vi "UsrProfiles-Selective save.vi"(11 "Changes array ctrl":refnum<vi>) -> (0 "error out":errorcluster)   [LabVIEW 2017]
uses:
  Typedefs/Which path.ctl
  <vilib>/Utility/config.llb/NI_LVConfig.lvlib
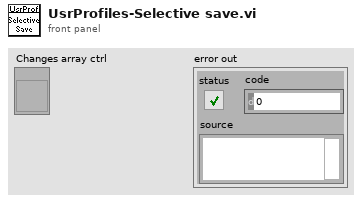
[diagram p1: front panel]
types:
  T1 = typedef "Changes info cluster-DBL.ctl" = cluster{"Section names":string[], "Keys data":T2}
  T2 = typedef "Ini file interface (DBL).ctl" = cluster{"key":string, "Save?":bool, "Default":dbl}[]
  T3 = typedef "Changes info cluster-STRING.ctl" = cluster{"Section names":string[], "Keys data":T4}
  T4 = typedef "Ini file interface (String).ctl" = cluster{"key":string, "Save?":bool, "Default":string}[]
  T5 = typedef "Changes info cluster-BOOL.ctl" = cluster{"Section names":string[], "Keys data":T6}
  T6 = typedef "Ini file interface (Boolean).ctl" = cluster{"key":string, "Save?":bool, "Default":bool}[]
  T7 = typedef "Which path.ctl" = enum16{"Configuration Files", "Calibration Files", "Images", "Setup.ini", "Loaded User profile.ini", "User's-Previous session.ini", "New user profile.ini", "Selected User profile.ini", "User profiles folder", "Power meter scaling.txt", "FOV Cal.ini"}
  T8 = typedef "NI_LVConfig.lvlib/Config Data RefNum.ctl" = refnum<k1>
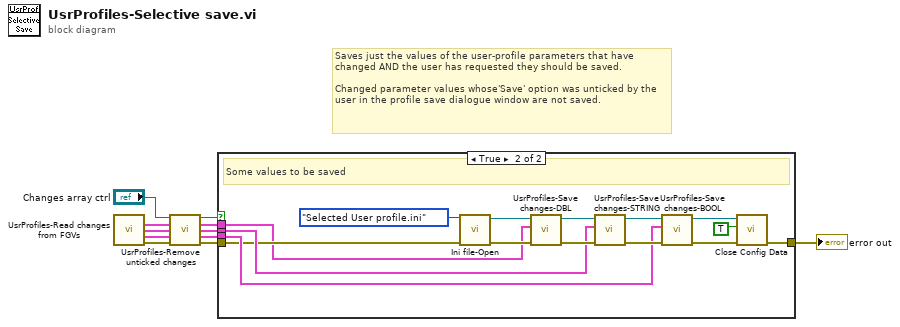
[diagram p0: block diagram]
diagram:
  # "Saves just the values of the user-profile parameters that have changed AND the user has requested they should be saved.\n\nChanged parameter values whose'Save' option was unticked by the user in the profile save dialogue window are not saved."
  n1 = call "UsrProfiles-Read changes from FGVs.vi"() -> ("Keys of changed parameters-DBL"=w9:T1, "Keys of changed parameters-STRING"=w8:T3, "Keys of changed parameters-BOOL"=w7:T5, "error out"=w11:errorcluster)  [unwired: 10 in, 2 out]
  n2 = call "UsrProfiles-Remove unticked changes.vi"("Changes array ctrl"="Changes array ctrl", "Keys of changed parameters-DBL"=w9, "Keys of changed parameters-STRING"=w8, "Keys of changed parameters-BOOL"=w7, "error in (no error)"=w11) -> ("Some values to be saved"=w2:bool, "Keys of changed parameters-DBL"=w3:T1, "Keys of changed parameters-STRING"=w6:T3, "Keys of changed parameters-BOOL"=w5:T5, "error out"=w4:errorcluster)  [unwired: 6 in]
  n3 = case shown="True" w2 {
    tunnel: w6 -> [_ w18]
    tunnel: w5 -> [_ w17]
    tunnel: [w12 w16] -> w1
    tunnel: w4 -> [w12 w14]
    tunnel: w3 -> [_ w13]
    frame False {
      # "No values to be saved"
    }
    frame True {
      # "Some values to be saved"
      n4 = call "Ini file-Open.vi"("Error In"=w14, "Which file?"=Which_path."Selected User profile.ini" ("Which file? (User profile.ini)")) -> ("error out"=w15:errorcluster, "User profile ini file ref"=w25:T8)  [unwired: 6 in, 2 out]
      n5 = call "UsrProfiles-Save changes-DBL.vi"("error in (no error)"=w15, "Keys of changed parameters-DBL"=w13, "User profile ini file ref"=w25) -> ("error out"=w21:errorcluster, "User profile ini file ref"=w24:T8)  [unwired: 7 in]
      n6 = call "UsrProfiles-Save changes-STRING.vi"("error in (no error)"=w21, "Keys of changed parameters-STRING"=w18, "User profile ini file ref"=w24) -> ("error out"=w22:errorcluster, "User profile ini file ref"=w23:T8)  [unwired: 7 in]
      n7 = call "UsrProfiles-Save changes-BOOL.vi"("error in (no error)"=w22, "Keys of changed parameters-BOOL"=w17, "User profile ini file ref"=w23) -> ("error out"=w19:errorcluster, "User profile ini file ref"=w20:T8)  [unwired: 7 in]
      n8 = call <vilib>:"Close Config Data.vi"("error in (no error)"=w19, "write file if changed (T)"=TRUE ("write configuration file? (F)"), "refnum"=w20) -> ("error out"=w16:errorcluster)  [unwired: 7 in, 1 out]
    }
  }
  "error out" <- w1
